vi "1553ICD Test.vi"() -> ()   [LabVIEW 2020]
uses:
  user.lib/18s-File-Operation/File-EXP/Typedef/Def-File-EXP.ctl
  user.lib/18s-File-Operation/File-EXP/File-EXP.lvlib
  MAL-ServoProduct/MAL-ServoProduct.lvclass
  user.lib/_LVAPT/1553ICD/1553-ICD.lvlib
panel:
  out "error out":errorcluster
  out "波形图 3":dbl[](graph)
  in  "禁用的索引 (列) 3":i32
  out "数组 4":string[](array[string])
  out "转换数据(U16)":u16[][](array[numeric]) format="%.0x"
  in  "禁用的索引 (列) 2":i32
  out "波形图 2":dbl[](graph)
  in  "禁用的索引 (列)":i32
  out "波形图":u16[](graph)
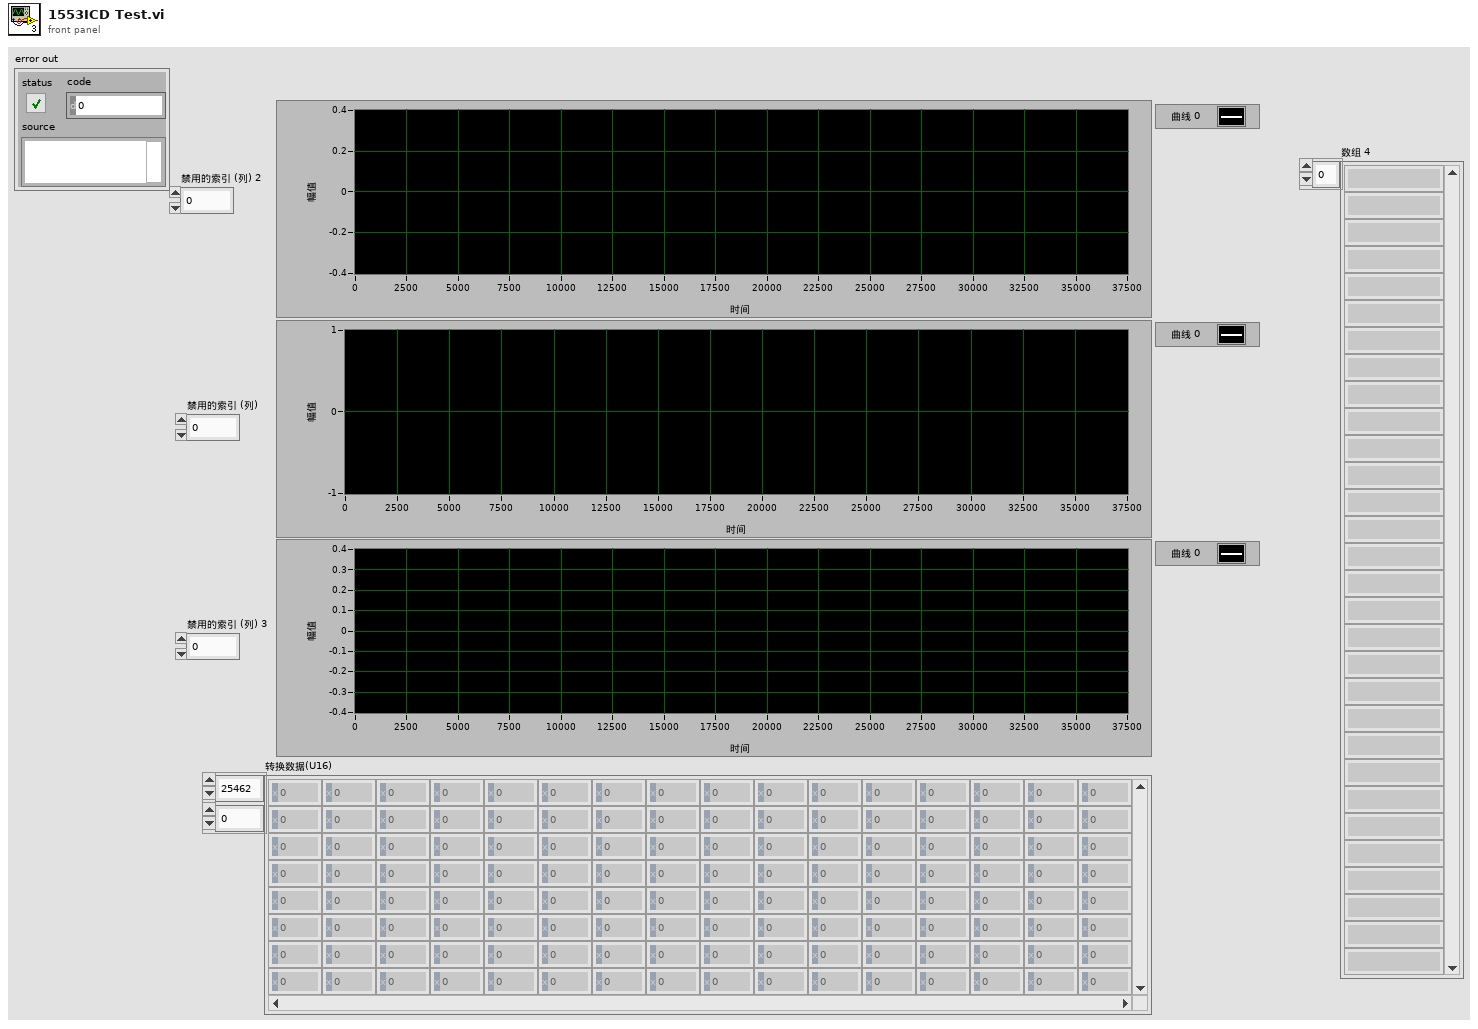
[diagram p1: front panel]
types:
  T1 = typedef "File-EXP.lvlib/Def-File-EXP.ctl" = cluster{"EXP-Header":cluster{"Token":string, "Version":string, "Name":string, "ConfigurationList":cluster{"Name":string, "Value":string}[]}, "ItemList":cluster{"Name":string, "Value":string}[]}
  T2 = cluster{"FileName":string, "AI CfgMap":variant, "1553 解码 CfgMap":variant, "1553 编码 CfgMap":variant}
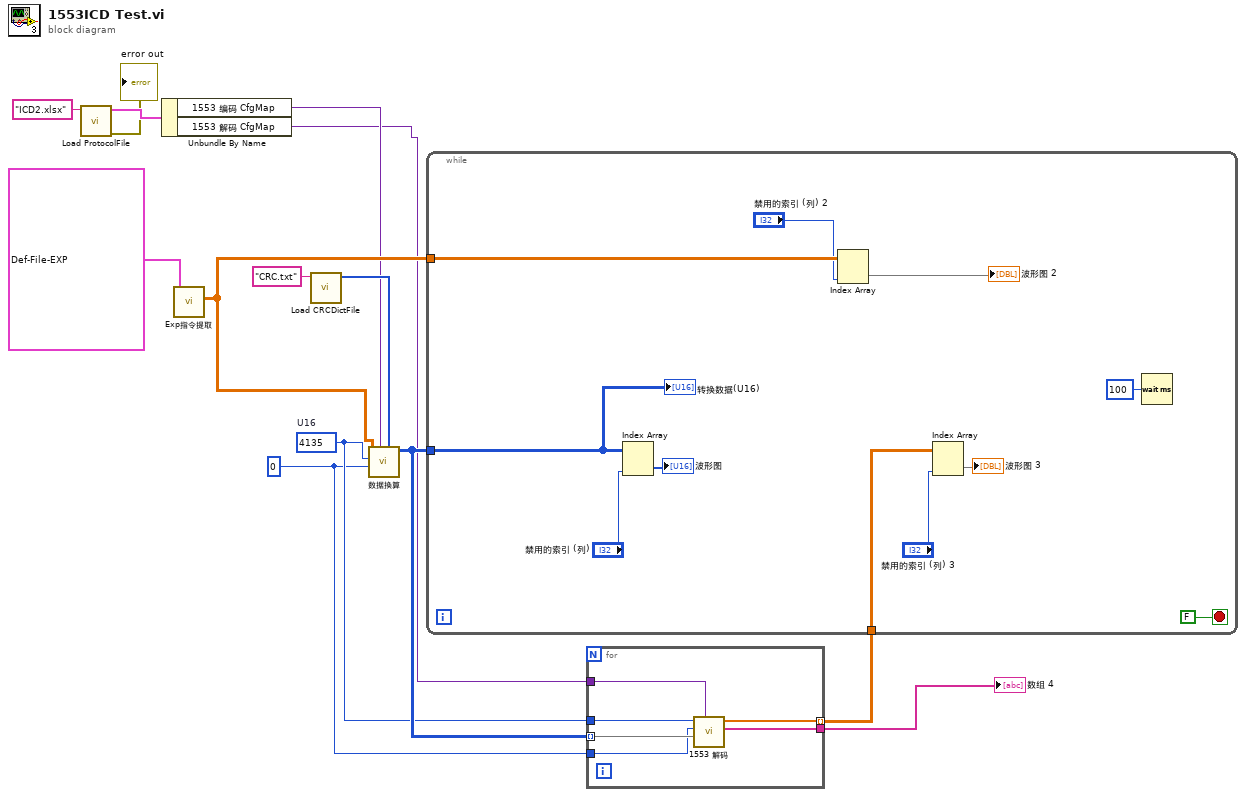
[diagram p0: block diagram]
diagram:
  w6 = u16 4135  # U16
  w5 = u16 0 ("CMD2")
  n1 = call "Load ProtocolFile.vi"("pattern"="ICD2.xlsx") -> ("error out"=→"error out":errorcluster, "ProtocolFile"=w9:T2)  [unwired: 9 in]
  n2 = Unbundle By Name(w9) -> ("1553 编码 CfgMap"=w8:variant, "1553 解码 CfgMap"=w4:variant)
  n3 = call "Exp指令提取.vi"("Def-File-EXP"=T1 {"EXP-Header"={"Token"="TestExpress", "Version"="", "Name"="II作动器频率特性测试", "ConfigurationList"=[{"Name"="HC_FLAG", "Value"="0"}, {"Name"="PRO", "Value"="1K27-31B_ereqa_A.pro"}, {"Name"="STD", "Value"="1K27-31B_danji.std"}, {"Name"="数据发送点数/秒", "Value"="1000"}, {"Name"="数据采集点数/秒", "Value"="1000"}, {"Name"="数字通讯采样率", "Value"="1000"}, {"Name"="", "Value"=""}, {"Name"="TDMS文件名称", "Value"="II作动器频率特性测试.tdms"}, {"Name"="EXP版本号", "Value"="v1.0"}, {"Name"="硬件描述文件", "Value"="servo_product2.hw"}, {"Name"="通道分配信息", "Value"="DAQAI(4) 1553(39)"}, {"Name"="", "Value"=""}, {"Name"="1553Channel", "Value"="1553ChannelA"}, {"Name"="InterruptCmdLength", "Value"="1000"}, {"Name"="InterruptNum", "Value"="10"}, {"Name"="BCCMDArray", "Value"="0x1027 0x142B 0x1455"}, {"Name"="CMDGapTime", "Value"="200 300 500"}, {"Name"="", "Value"=""}, {"Name"="DAQAIDevice", "Value"="NI6363A"}, {"Name"="", "Value"=""}, {"Name"="DAQAODevice", "Value"=""}]}, "ItemList"=[{"Name"="STD_V/A", "Value"="-4.5"}, {"Name"="BOARD_NUM", "Value"="2"}, {"Name"="V/A_NUM", "Value"="4"}, {"Name"="ACT_V/A", "Value"="4.9839   4.9862    5.0199    5.0597"}, {"Name"="STARTTIME", "Value"="0"}, {"Name"="ALL_CHANNEL_NAME", "Value"="43\r角位移A      角位移B      角位移C      角位移D\r时标高1      时标低1      作动器I指令        作动器II指令\r作动器III指令        作动器IV指令         CRC1            时标高2\r时标低2       作动器I位移        作动器II位移             作动器III位移\r作动器IV位移     Iq电流I       Iq电流II          Iq电流III\rIq电流IV         160V          时标高3           时标低3\rId电流I          Id电流II      Id电流III         Id电流IV\rIu电流I          Iu电流II      Iu电流III         Iu电流IV\rIv电流I          Iv电流II      Iv电流III         Iv电流IV\r电机转速I        电机转速II    电机转速III        电机转速IV\rCRC出错总次数    总线协议芯片出错总次数              看门狗复位总次数"}, {"Name"="ACQ_CHANNEL", "Value"="1 2 3 4 5 6 7 8 9 10 11 12 13 14 15 16\r17 18 19 20 21 22 23 24 25 26 27 28 29 30 31 32"}, {"Name"="DISP_CHANNEL_NUM", "Value"="12"}, {"Name"="DISP_CHANNEL", "Value"="1 2 3 4 5 6 7 8 13 14 15 16"}, {"Name"="DISP_COLOR", "Value"="255 0 0  255 255 0  0 0 255  255 255 255  128 0 0  0 128 0  0 0 128  128 128 0\r0 255 255  255 128 0  255 0 255  128 0 255"}, {"Name"="ResponseNum", "Value"="42\r0 21 21 1 1K27-31B_Freqa045_A.dat 频率特性 0.45° 0\r1  9997  9.4340 2000  0 0 0 0 1 0 ah2_0015.bin 频率特性 0.159Hz,0.45° 50316 100628 0 0\r信号1  2  0.159 1.552  0.0  0 0 0 0   0    0    0.0  0   0.0  0   频率特性,0.45°3T\r信号1  0  1  0.0 0.0  0 0 0 0   0    0    0.0  0   0.0  0   零位\r信号1  0  1  0.0 0.0  0 0 0 0   0    0    0.0  0   0.0  0   零位\r信号1  0  1  0.0 0.0  0 0 0 0   0    0    0.0  0   0.0  0   零位\r2  9997  0.40 1000  0 0 0 0 0 0 ZeroF-1.bin 零位 0v 100 1000 0 0\r信号1  0  1  0.0 0.0  0 0 0 0   0    0    0.0  0   0.0  0   零位\r信号1  0  1  0.0 0.0  0 0 0 0   0    0    0.0  0   0.0  0   零位\r信号1  0  1  0.0 0.0  0 0 0 0   0    0    0.0  0   0.0  0   零位\r信号1  0  1  0.0 0.0  0 0 0 0   0    0    0.0  0   0.0  0   零位\r3  9997  3  2000  0 0 0 0 1 0 ah2_0100.bin 频率特性 1.000Hz,0.45° 8002 16000 0 0\r信号1  2  1.000 1.552   0.0  0 0 0 0   0    0    0.0  0   0.0  0   频率特性,0.45°3T\r信号1  0  1  0.0 0.0  0 0 0 0   0    0    0.0  0   0.0  0   零位\r信号1  0  1  0.0 0.0  0 0 0 0   0    0    0.0  0   0.0  0   零位\r信号1  0  1  0.0 0.0  0 0 0 0   0    0    0.0  0   0.0  0   零位\r4  9997  0.40 1000  0 0 0 0 0 0 ZeroF-2.bin 零位 0v 100 1000 0 0\r信号1  0  1  0.0 0.0  0 0 0 0   0    0    0.0  0   0.0  0   零位\r信号1  0  1  0.0 0.0  0 0 0 0   0    0    0.0  0   0.0  0   零位\r信号1  0  1  0.0 0.0  0 0 0 0   0    0    0.0  0   0.0  0   零位\r信号1  0  1  0.0 0.0  0 0 0 0   0    0    0.0  0   0.0  0   零位\r5  9997  1.8844  4000  0 0 0 0 1 0 ah2_0159.bin 频率特性 1.592Hz,0.45° 5024 10044 0 0\r信号1  2  1.592 1.552   0.0  0 0 0 0   0    0    0.0  0   0.0  0   频率特性,0.45°3T\r信号1  0  1  0.0 0.0  0 0 0 0   0    0    0.0  0   0.0  0   零位\r信号1  0  1  0.0 0.0  0 0 0 0   0    0    0.0  0   0.0  0   零位\r信号1  0  1  0.0 0.0  0 0 0 0   0    0    0.0  0   0.0  0   零位\r6  9997  0.40 1000  0 0 0 0 0 0 ZeroF-3.bin 零位 0v 100 1000 0 0\r信号1  0  1  0.0 0.0  0 0 0 0   0    0    0.0  0   0.0  0   零位\r信号1  0  1  0.0 0.0  0 0 0 0   0    0    0.0  0   0.0  0   零位\r信号1  0  1  0.0 0.0  0 0 0 0   0    0    0.0  0   0.0  0   零位\r信号1  0  1  0.0 0.0  0 0 0 0   0    0    0.0  0   0.0  0   零位\r7  9997  1.256  6000  0 0 0 0 1 0 ah2_0238.bin 频率特性  2.387Hz,0.45° 3352 6700 0 0\r信号1  2  2.387 1.552 0.0  0 0 0 0   0    0    0.0  0   0.0  0   频率特性,0.45°3T\r信号1  0  1  0.0 0.0  0 0 0 0   0    0    0.0  0   0.0  0   零位\r信号1  0  1  0.0 0.0  0 0 0 0   0    0    0.0  0   0.0  0   零位\r信号1  0  1  0.0 0.0  0 0 0 0   0    0    0.0  0   0.0  0   零位\r8  9997  0.40 1000  0 0 0 0 0 0 ZeroF-4.bin 零位 0v 100 1000 0 0\r信号1  0  1  0.0 0.0  0 0 0 0   0    0    0.0  0   0.0  0   零位\r信号1  0  1  0.0 0.0  0 0 0 0   0    0    0.0  0   0.0  0   零位\r信号1  0  1  0.0 0.0  0 0 0 0   0    0    0.0  0   0.0  0   零位\r信号1  0  1  0.0 0.0  0 0 0 0   0    0    0.0  0   0.0  0   零位\r9  9997  0.9425  6000  0 0 0 0 1 0 ah2_0318.bin 频率特性   3.183Hz,0.45° 2514 5023 0 0\r信号1  2  3.183 1.552 0.0  0 0 0 0   0    0    0.0  0   0.0  0   频率特性,0.45°3T\r信号1  0  1  0.0 0.0  0 0 0 0   0    0    0.0  0   0.0  0   零位\r信号1  0  1  0.0 0.0  0 0 0 0   0    0    0.0  0   0.0  0   零位\r信号1  0  1  0.0 0.0  0 0 0 0   0    0    0.0  0   0.0  0   零位\r10  9997  0.40 1000  0 0 0 0 0 0 ZeroF-5.bin 零位 0v 100 1000 0 0\r信号1  0  1  0.0 0.0  0 0 0 0   0    0    0.0  0   0.0  0   零位\r信号1  0  1  0.0 0.0  0 0 0 0   0    0    0.0  0   0.0  0   零位\r信号1  0  1  0.0 0.0  0 0 0 0   0    0    0.0  0   0.0  0   零位\r信号1  0  1  0.0 0.0  0 0 0 0   0    0    0.0  0   0.0  0   零位\r11  9997  0.62827 6000  0 0 0 0 1 0 ah2_0477.bin 频率特性   4.775Hz,0.45° 1676 3349 0 0\r信号1  2  4.775 1.552 0.0  0 0 0 0   0    0    0.0  0   0.0  0   频率特性,0.45°3T\r信号1  0  1  0.0 0.0  0 0 0 0   0    0    0.0  0   0.0  0   零位\r信号1  0  1  0.0 0.0  0 0 0 0   0    0    0.0  0   0.0  0   零位\r信号1  0  1  0.0 0.0  0 0 0 0   0    0    0.0  0   0.0  0   零位\r12  9997  0.40 1000  0 0 0 0 0 0 ZeroF-6.bin 零位 0v 100 1000 0 0\r信号1  0  1  0.0 0.0  0 0 0 0   0    0    0.0  0   0.0  0   零位\r信号1  0  1  0.0 0.0  0 0 0 0   0    0    0.0  0   0.0  0   零位\r信号1  0  1  0.0 0.0  0 0 0 0   0    0    0.0  0   0.0  0   零位\r信号1  0  1  0.0 0.0  0 0 0 0   0    0    0.0  0   0.0  0   零位\r13  9997  0.9425 6000  0 0 0 0 1 0 ah2_0636.bin 频率特性   6.366Hz,0.45° 1257 5024 0 0\r信号1  2  6.366 1.552 0.0  0 0 0 0   0    0    0.0  0   0.0  0   频率特性,0.45°6T\r信号1  0  1  0.0 0.0  0 0 0 0   0    0    0.0  0   0.0  0   零位\r信号1  0  1  0.0 0.0  0 0 0 0   0    0    0.0  0   0.0  0   零位\r信号1  0  1  0.0 0.0  0 0 0 0   0    0    0.0  0   0.0  0   零位\r14  9997  0.40 1000  0 0 0 0 0 0 ZeroF-6.bin 零位 0v 100 1000 0 0\r信号1  0  1  0.0 0.0  0 0 0 0   0    0    0.0  0   0.0  0   零位\r信号1  0  1  0.0 0.0  0 0 0 0   0    0    0.0  0   0.0  0   零位\r信号1  0  1  0.0 0.0  0 0 0 0   0    0    0.0  0   0.0  0   零位\r信号1  0  1  0.0 0.0  0 0 0 0   0    0    0.0  0   0.0  0   零位\r15  9997  0.7540 6000  0 0 0 0 1 0 ah2_0795.bin 频率特性   7.958Hz,0.45° 1005 4019 0 0\r信号1  2  7.958 1.552 0.0  0 0 0 0   0    0    0.0  0   0.0  0   频率特性,0.45°6T\r信号1  0  1  0.0 0.0  0 0 0 0   0    0    0.0  0   0.0  0   零位\r信号1  0  1  0.0 0.0  0 0 0 0   0    0    0.0  0   0.0  0   零位\r信号1  0  1  0.0 0.0  0 0 0 0   0    0    0.0  0   0.0  0   零位\r16  9997  0.40 1000  0 0 0 0 0 0 ZeroF-7.bin 零位 0v 100 1000 0 0\r信号1  0  1  0.0 0.0  0 0 0 0   0    0    0.0  0   0.0  0   零位\r信号1  0  1  0.0 0.0  0 0 0 0   0    0    0.0  0   0.0  0   零位\r信号1  0  1  0.0 0.0  0 0 0 0   0    0    0.0  0   0.0  0   零位\r信号1  0  1  0.0 0.0  0 0 0 0   0    0    0.0  0   0.0  0   零位\r17  9997 0.6283 6000  0 0 0 0 1 0 ah2_0954.bin 频率特性   9.549Hz,0.45° 838 3349 0 0\r信号1  2  9.549 1.552 0.0  0 0 0 0   0    0    0.0  0   0.0  0   频率特性,0.45°6T\r信号1  0  1  0.0 0.0  0 0 0 0   0    0    0.0  0   0.0  0   零位\r信号1  0  1  0.0 0.0  0 0 0 0   0    0    0.0  0   0.0  0   零位\r信号1  0  1  0.0 0.0  0 0 0 0   0    0    0.0  0   0.0  0   零位\r18  9997  0.40 1000  0 0 0 0 0 0 ZeroF-8.bin 零位 0v 100 1000 0 0\r信号1  0  1  0.0 0.0  0 0 0 0   0    0    0.0  0   0.0  0   零位\r信号1  0  1  0.0 0.0  0 0 0 0   0    0    0.0  0   0.0  0   零位\r信号1  0  1  0.0 0.0  0 0 0 0   0    0    0.0  0   0.0  0   零位\r信号1  0  1  0.0 0.0  0 0 0 0   0    0    0.0  0   0.0  0   零位\r19  9997  0.897  6000  0 0 0 0 1 0 ah2_1114.bin 频率特性   11.14Hz,0.45° 2154 4306 0 0\r信号1  2  11.14   1.552 0.0  0 0 0 0   0    0    0.0  0   0.0  0   频率特性,0.45°10T\r信号1  0  1  0.0 0.0  0 0 0 0   0    0    0.0  0   0.0  0   零位\r信号1  0  1  0.0 0.0  0 0 0 0   0    0    0.0  0   0.0  0   零位\r信号1  0  1  0.0 0.0  0 0 0 0   0    0    0.0  0   0.0  0   零位\r20  9997  0.40 1000  0 0 0 0 0 0 ZeroF-5.bin 零位 0v 100 1000 0 0\r信号1  0  1  0.0 0.0  0 0 0 0   0    0    0.0  0   0.0  0   零位\r信号1  0  1  0.0 0.0  0 0 0 0   0    0    0.0  0   0.0  0   零位\r信号1  0  1  0.0 0.0  0 0 0 0   0    0    0.0  0   0.0  0   零位\r信号1  0  1  0.0 0.0  0 0 0 0   0    0    0.0  0   0.0  0   零位\r21  9996  0.7855  6000  0 0 0 0 1 0 ah2_1273.bin 频率特性   12.73Hz,0.45° 1885 3768 0 0\r信号1  2   12.73   1.552 0.0  0 0 0 0   0    0    0.0  0   0.0  0   频率特性,0.45°10T\r信号1  0  1  0.0 0.0  0 0 0 0   0    0    0.0  0   0.0  0   零位\r信号1  0  1  0.0 0.0  0 0 0 0   0    0    0.0  0   0.0  0   零位\r信号1  0  1  0.0 0.0  0 0 0 0   0    0    0.0  0   0.0  0   零位\r22  9996  0.40 1000  0 0 0 0 0 0 ZeroF-5.bin 零位 0v 100 1000 0 0\r信号1  0  1  0.0 0.0  0 0 0 0   0    0    0.0  0   0.0  0   零位\r信号1  0  1  0.0 0.0  0 0 0 0   0    0    0.0  0   0.0  0   零位\r信号1  0  1  0.0 0.0  0 0 0 0   0    0    0.0  0   0.0  0   零位\r信号1  0  1  0.0 0.0  0 0 0 0   0    0    0.0  0   0.0  0   零位\r23  9996  0.698  6000  0 0 0 0 1 0 ah2_1432.bin 频率特性   14.32Hz,0.45° 1676 3350 0 0\r信号1  2  14.32 1.552 0.0  0 0 0 0   0    0    0.0  0   0.0  0   频率特性,0.45°10T\r信号1  0  1  0.0 0.0  0 0 0 0   0    0    0.0  0   0.0  0   零位\r信号1  0  1  0.0 0.0  0 0 0 0   0    0    0.0  0   0.0  0   零位\r信号1  0  1  0.0 0.0  0 0 0 0   0    0    0.0  0   0.0  0   零位\r24  9996  0.40 1000  0 0 0 0 0 0 ZeroF-5.bin 零位 0v 100 1000 0 0\r信号1  0  1  0.0 0.0  0 0 0 0   0    0    0.0  0   0.0  0   零位\r信号1  0  1  0.0 0.0  0 0 0 0   0    0    0.0  0   0.0  0   零位\r信号1  0  1  0.0 0.0  0 0 0 0   0    0    0.0  0   0.0  0   零位\r信号1  0  1  0.0 0.0  0 0 0 0   0    0    0.0  0   0.0  0   零位\r25  9996  0.7537  6000  0 0 0 0 1 0 ah2_1592.bin 频率特性   15.92Hz,0.45° 1507 4018 0 0\r信号1  2  15.92 1.552 0.0  0 0 0 0   0    0    0.0  0   0.0  0   频率特性,0.45°12T\r信号1  0  1  0.0 0.0  0 0 0 0   0    0    0.0  0   0.0  0   零位\r信号1  0  1  0.0 0.0  0 0 0 0   0    0    0.0  0   0.0  0   零位\r信号1  0  1  0.0 0.0  0 0 0 0   0    0    0.0  0   0.0  0   零位\r26  9996  0.40 1000  0 0 0 0 0 0 ZeroF-5.bin 零位 0v 100 1000 0 0\r信号1  0  1  0.0 0.0  0 0 0 0   0    0    0.0  0   0.0  0   零位\r信号1  0  1  0.0 0.0  0 0 0 0   0    0    0.0  0   0.0  0   零位\r信号1  0  1  0.0 0.0  0 0 0 0   0    0    0.0  0   0.0  0   零位\r信号1  0  1  0.0 0.0  0 0 0 0   0    0    0.0  0   0.0  0   零位\r27  9996  0.628  6000  0 0 0 0 1 0 ah2_1910.bin 频率特性   19.10Hz,0.45° 1256 3349 0 0\r信号1  2  19.10 1.552 0.0  0 0 0 0   0    0    0.0  0   0.0  0   频率特性,0.45°12T\r信号1  0  1  0.0 0.0  0 0 0 0   0    0    0.0  0   0.0  0   零位\r信号1  0  1  0.0 0.0  0 0 0 0   0    0    0.0  0   0.0  0   零位\r信号1  0  1  0.0 0.0  0 0 0 0   0    0    0.0  0   0.0  0   零位\r28  9996  0.40 1000  0 0 0 0 0 0 ZeroF-5.bin 零位 0v 100 1000 0 0\r信号1  0  1  0.0 0.0  0 0 0 0   0    0    0.0  0   0.0  0   零位\r信号1  0  1  0.0 0.0  0 0 0 0   0    0    0.0  0   0.0  0   零位\r信号1  0  1  0.0 0.0  0 0 0 0   0    0    0.0  0   0.0  0   零位\r信号1  0  1  0.0 0.0  0 0 0 0   0    0    0.0  0   0.0  0   零位\r29  9996  0.897 6000  0 0 0 0 1 0 ah2_22.28.bin 频率特性   22.28Hz,0.45° 1796 5024 0 0\r信号1  2  22.28 1.552 0.0  0 0 0 0   0    0    0.0  0   0.0  0   频率特性,0.45°20T\r信号1  0  1  0.0 0.0  0 0 0 0   0    0    0.0  0   0.0  0   零位\r信号1  0  1  0.0 0.0  0 0 0 0   0    0    0.0  0   0.0  0   零位\r信号1  0  1  0.0 0.0  0 0 0 0   0    0    0.0  0   0.0  0   零位\r30  9996  0.40 1000  0 0 0 0 0 0 ZeroF-5.bin 零位 0v 100 1000 0 0\r信号1  0  1  0.0 0.0  0 0 0 0   0    0    0.0  0   0.0  0   零位\r信号1  0  1  0.0 0.0  0 0 0 0   0    0    0.0  0   0.0  0   零位\r信号1  0  1  0.0 0.0  0 0 0 0   0    0    0.0  0   0.0  0   零位\r信号1  0  1  0.0 0.0  0 0 0 0   0    0    0.0  0   0.0  0   零位\r31  9996  0.785  6000  0 0 0 0 1 0 ah2_25.47.bin 频率特性   25.47Hz,0.45° 1570 4395 0 0\r信号1  2  25.47 1.552 0.0  0 0 0 0   0    0    0.0  0   0.0  0   频率特性,0.45°20T\r信号1  0  1  0.0 0.0  0 0 0 0   0    0    0.0  0   0.0  0   零位\r信号1  0  1  0.0 0.0  0 0 0 0   0    0    0.0  0   0.0  0   零位\r信号1  0  1  0.0 0.0  0 0 0 0   0    0    0.0  0   0.0  0   零位\r32  9996  0.40 1000  0 0 0 0 0 0 ZeroF-5.bin 零位 0v 100 1000 0 0\r信号1  0  1  0.0 0.0  0 0 0 0   0    0    0.0  0   0.0  0   零位\r信号1  0  1  0.0 0.0  0 0 0 0   0    0    0.0  0   0.0  0   零位\r信号1  0  1  0.0 0.0  0 0 0 0   0    0    0.0  0   0.0  0   零位\r信号1  0  1  0.0 0.0  0 0 0 0   0    0    0.0  0   0.0  0   零位\r33  9996  0.698  6000  0 0 0 0 1 0 ah2_2865.bin 频率特性   28.65Hz,0.45° 1396 3907 0 0\r信号1  2  28.65 1.552 0.0  0 0 0 0   0    0    0.0  0   0.0  0   频率特性,0.45°20T\r信号1  0  1  0.0 0.0  0 0 0 0   0    0    0.0  0   0.0  0   零位\r信号1  0  1  0.0 0.0  0 0 0 0   0    0    0.0  0   0.0  0   零位\r信号1  0  1  0.0 0.0  0 0 0 0   0    0    0.0  0   0.0  0   零位\r34  9996  0.40 1000  0 0 0 0 0 0 ZeroF-5.bin 零位 0v 100 1000 0 0\r信号1  0  1  0.0 0.0  0 0 0 0   0    0    0.0  0   0.0  0   零位\r信号1  0  1  0.0 0.0  0 0 0 0   0    0    0.0  0   0.0  0   零位\r信号1  0  1  0.0 0.0  0 0 0 0   0    0    0.0  0   0.0  0   零位\r信号1  0  1  0.0 0.0  0 0 0 0   0    0    0.0  0   0.0  0   零位\r35  9996  0.6283  6000  0 0 0 0 1 0 ah2_3183.bin 频率特性   31.83Hz,0.45° 1257 3517 0 0\r信号1  2  31.83 1.552 0.0  0 0 0 0   0    0    0.0  0   0.0  0   频率特性,0.45°20T\r信号1  0  1  0.0 0.0  0 0 0 0   0    0    0.0  0   0.0  0   零位\r信号1  0  1  0.0 0.0  0 0 0 0   0    0    0.0  0   0.0  0   零位\r信号1  0  1  0.0 0.0  0 0 0 0   0    0    0.0  0   0.0  0   零位\r36  9996  0.40 1000  0 0 0 0 0 0 ZeroF-5.bin 零位 0v 100 1000 0 0\r信号1  0  1  0.0 0.0  0 0 0 0   0    0    0.0  0   0.0  0   零位\r信号1  0  1  0.0 0.0  0 0 0 0   0    0    0.0  0   0.0  0   零位\r信号1  0  1  0.0 0.0  0 0 0 0   0    0    0.0  0   0.0  0   零位\r信号1  0  1  0.0 0.0  0 0 0 0   0    0    0.0  0   0.0  0   零位\r37  9996  0.914  6000  0 0 0 0 1 0 ah2_3500.bin 频率特性   35.00Hz,0.45° 1600  5482 0 0\r信号1  2  35.00 1.552 0.0  0 0 0 0   0    0    0.0  0   0.0  0   频率特性,0.45°32T\r信号1  0  1  0.0 0.0  0 0 0 0   0    0    0.0  0   0.0  0   零位\r信号1  0  1  0.0 0.0  0 0 0 0   0    0    0.0  0   0.0  0   零位\r信号1  0  1  0.0 0.0  0 0 0 0   0    0    0.0  0   0.0  0   零位\r38  9996  0.40 1000  0 0 0 0 0 0 ZeroF-5.bin 零位 0v 100 1000 0 0\r信号1  0  1  0.0 0.0  0 0 0 0   0    0    0.0  0   0.0  0   零位\r信号1  0  1  0.0 0.0  0 0 0 0   0    0    0.0  0   0.0  0   零位\r信号1  0  1  0.0 0.0  0 0 0 0   0    0    0.0  0   0.0  0   零位\r信号1  0  1  0.0 0.0  0 0 0 0   0    0    0.0  0   0.0  0   零位\r39  9996  0.966  6000  0 0 0 0 1 0 ah2_4138.bin 频率特性   41.38Hz,0.45° 1740 4796 0 0\r信号1  2  41.38  1.552 0.0  0 0 0 0   0    0    0.0  0   0.0  0   频率特性,0.45°40T\r信号1  0  1  0.0 0.0  0 0 0 0   0    0    0.0  0   0.0  0   零位\r信号1  0  1  0.0 0.0  0 0 0 0   0    0    0.0  0   0.0  0   零位\r信号1  0  1  0.0 0.0  0 0 0 0   0    0    0.0  0   0.0  0   零位\r40  9996  0.40 1000  0 0 0 0 0 0 ZeroF-5.bin 零位 0v 100 1000 0 0\r信号1  0  1  0.0 0.0  0 0 0 0   0    0    0.0  0   0.0  0   零位\r信号1  0  1  0.0 0.0  0 0 0 0   0    0    0.0  0   0.0  0   零位\r信号1  0  1  0.0 0.0  0 0 0 0   0    0    0.0  0   0.0  0   零位\r信号1  0  1  0.0 0.0  0 0 0 0   0    0    0.0  0   0.0  0   零位\r41  9996  0.897  6000  0 0 0 0 1 0 ah2_4458.bin 频率特性   44.585Hz,0.45° 1616 5381 0 0\r信号1  2  44.585  1.552 0.0  0 0 0 0   0    0    0.0  0   0.0  0   频率特性,0.45°40T\r信号1  0  1  0.0 0.0  0 0 0 0   0    0    0.0  0   0.0  0   零位\r信号1  0  1  0.0 0.0  0 0 0 0   0    0    0.0  0   0.0  0   零位\r信号1  0  1  0.0 0.0  0 0 0 0   0    0    0.0  0   0.0  0   零位\r42  9996  0.40 1000  0 0 0 0 0 0 ZeroF-6.bin 零位 0v 100 1000 0 0\r信号1  0  1  0.0 0.0  0 0 0 0   0    0    0.0  0   0.0  0   零位\r信号1  0  1  0.0 0.0  0 0 0 0   0    0    0.0  0   0.0  0   零位\r信号1  0  1  0.0 0.0  0 0 0 0   0    0    0.0  0   0.0  0   零位\r信号1  0  1  0.0 0.0  0 0 0 0   0    0    0.0  0   0.0  0   零位"}]} ("ConfigFile.EXP")) -> ("instruction data"=w13:dbl[][])  [unwired: 7 in, 3 out]
  n4 = call "Load CRCDictFile.vi"("Value"="CRC.txt") -> ("Array"=w12:u16[])  [unwired: 8 in, 2 out]
  n5 = call "数据换算.vi"("crc表格数据"=w12, "ConfigFile.ProtocolFile.1553 编码 CfgMap"=w8, "CMD2"=w5, "CMD1"=w6, "数据2D"=w13) -> ("转换数据(U16)"=w7:u16[][])  [unwired: 5 in, 1 out]
  n6 = for {
    tunnel: w7 -> [w20] mode=indexing
    tunnel: w6 -> [w19]
    tunnel: w5 -> [w18]
    tunnel: w4 -> [w17]
    tunnel: [w16] -> w2 mode=indexing
    tunnel: [w15] -> w3
    n7 = call "1553 解码.vi"("ConfigMap"=w17, "payload"=w20, "CMD2"=w18, "CMD1"=w19) -> ("数组 4"=w15:string[], "数组 3"=w16:dbl[])  [unwired: 5 in, 1 out]
  }
  "数组 4" <- w3
  n8 = while {
    tunnel: w13 -> [w27]
    tunnel: w7 -> [w24]
    tunnel: w2 -> [w21]
    stop <- FALSE stop-if-true
    n9 = Index Array(array=w24, index (col)="禁用的索引 (列)") -> (element=→"波形图":u16[])  [unwired: 1 in]
    n10 = Index Array(array=w27, index (col)="禁用的索引 (列) 2") -> (element=→"波形图 2":dbl[])  [unwired: 1 in]
    n11 = Index Array(array=w21, index (col)="禁用的索引 (列) 3") -> (element=→"波形图 3":dbl[])  [unwired: 1 in]
    n12 = Wait (ms)(milliseconds to wait=u32 100 ("等待时间（毫秒）")) -> ()  [unwired: 1 out]
    "转换数据(U16)" <- w24
  }
